vi "Send Command.vi"(4 "VISA Refnum in":refnum<visa-resource-name>, 6 "Motor On [Test]":bool, 7 "Receive Data?":bool, 8 "error in (no error)":errorcluster, 9 "Max Speed":u8, 10 "Steering Wheel [Test]":i8, 11 "Speed [Test]":i8) -> (0 "error out":errorcluster, 1 "output cluster":T1 {"Battery Level" scale=0.0..255.0})   [LabVIEW 2014]
uses:
  Controls/Controllers Clusters/Normal Operation Indicator Cluster.ctl
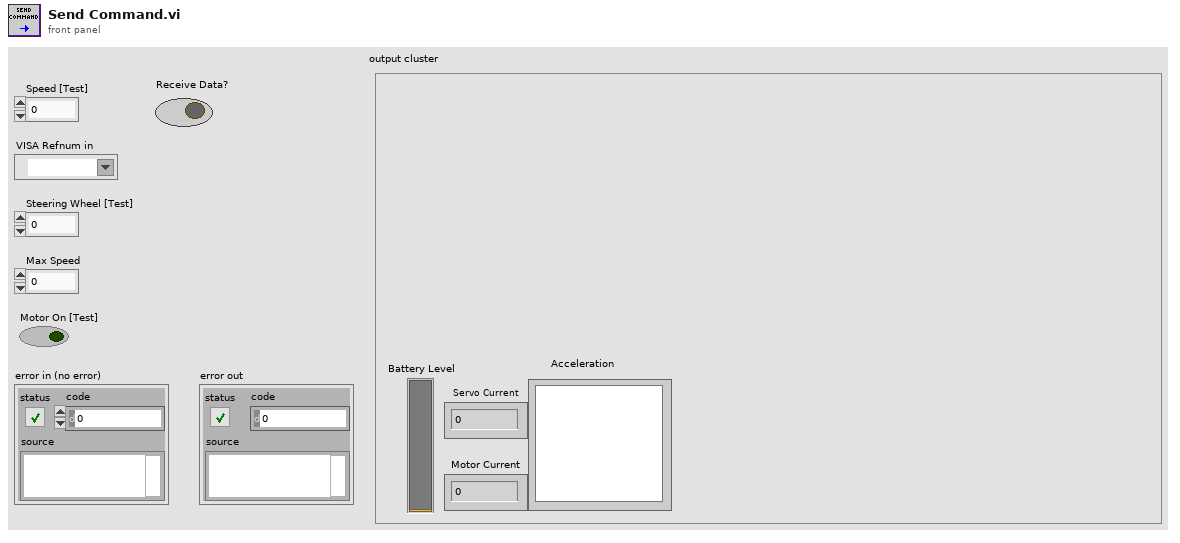
[diagram p1: front panel]
types:
  T1 = typedef "Normal Operation Indicator Cluster.ctl" = cluster{"Battery Level":u8, "Servo Current":dbl, "Motor Current":dbl, "Acceleration":cluster{"X":dbl, "Y":dbl}[]}
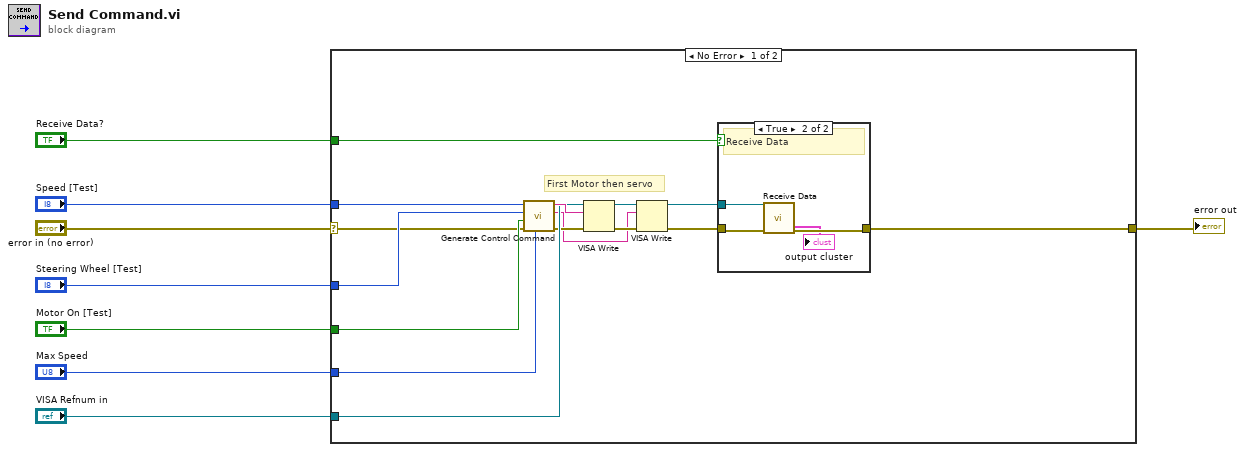
[diagram p0: block diagram]
diagram:
  n1 = case shown="No Error" "error in (no error)" {
    selector: "error in (no error)" -> [w16 w29]
    tunnel: "VISA Refnum in" -> [w22 _]
    tunnel: [w9 w29] -> w7
    tunnel: "Max Speed" -> [w20 _]
    tunnel: "Motor On [Test]" -> [w19 _]
    tunnel: "Steering Wheel [Test]" -> [w18 _]
    tunnel: "Speed [Test]" -> [w17 _]
    tunnel: "Receive Data?" -> [w11 _]
    frame No Error {
      # "First Motor then servo"
      n2 = call "Generate Control Command.vi"("Maximum Speed"=w20, "Error In"=w16, "Motor On"=w19, "Steering wheel"=w18, "Speed"=w17) -> ("Error Out"=w21:errorcluster, "Servo Command"=w13:string, "Motor Command"=w23:string)  [unwired: 4 in]
      n3 = VISA Write(VISA resource name=w22, write buffer=w23, error in (no error)=w21) -> (VISA resource name out=w14:refnum<visa-resource-name>, error out=w15:errorcluster)  [unwired: 1 out]
      n4 = VISA Write(VISA resource name=w14, write buffer=w13, error in (no error)=w15) -> (VISA resource name out=w12:refnum<visa-resource-name>, error out=w10:errorcluster)  [unwired: 1 out]
      n5 = case shown="True" w11 {
        tunnel: w12 -> [_ w26]
        tunnel: w10 -> [w24 w28]
        tunnel: [w24 w27] -> w9
        frame False {
          # "Don't receive data"
        }
        frame True {
          # "Receive Data"
          n6 = call "Receive Data.vi"("Error In"=w28, "VISA resource name"=w26) -> ("Error Out"=w27:errorcluster, "output cluster"=→"output cluster":T1)  [unwired: 8 in]
        }
      }
    }
    frame Error {
    }
  }
  "error out" <- w7
